vi "Build output file path.vi"(1 "Measurement type":string(combo), 2 "Current test directory":path) -> (0 "File path":path)   [LabVIEW 2018]
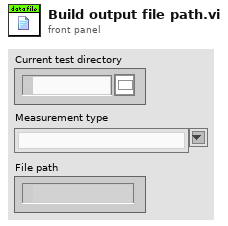
[diagram p1: front panel]
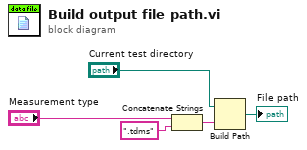
[diagram p0: block diagram]
diagram:
  n1 = Concatenate Strings("Measurement type", ".tdms" ("name or relative path")) -> (w1:string)
  n2 = Build Path(base path="Current test directory", name or relative path=w1) -> (appended path=→"File path":path)
